vi "Basic Example.vi"   [LabVIEW 2013, in "Progress Bar.lvlib"]
uses:
  Progress Bar.lvlib
  Controls/Update Bar Actions.ctl
types:
  T1 = typedef "Progress Bar.lvlib/Update Bar Actions.ctl" = enum16{"Add To Existing", "Set to Value"}
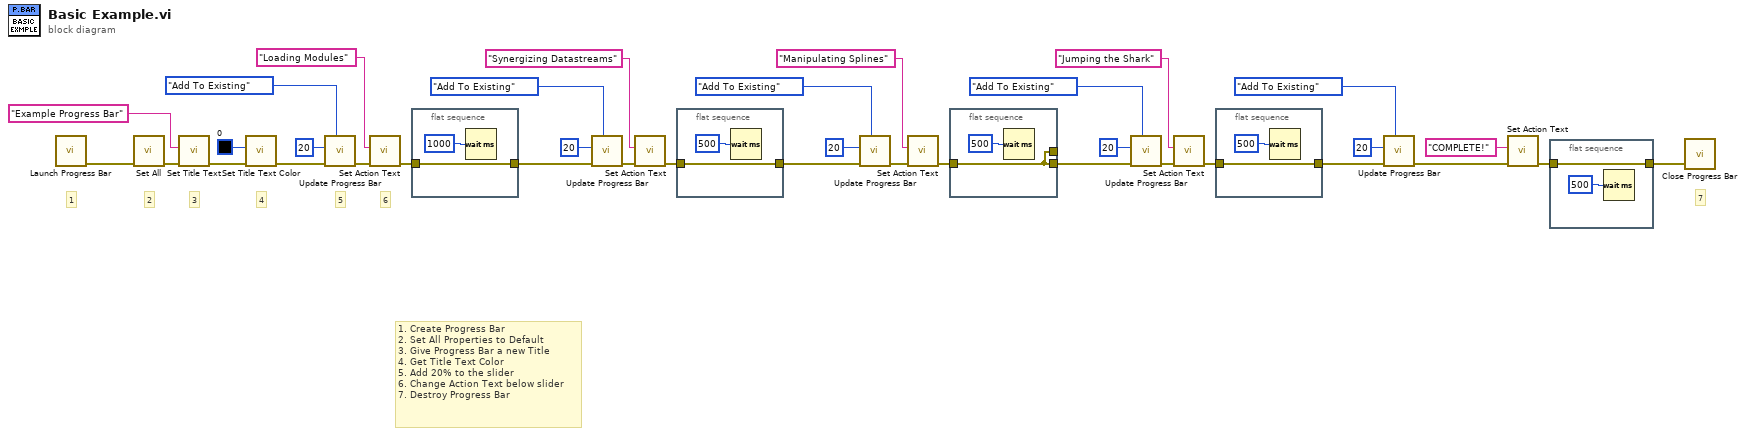
[diagram p0: block diagram]
diagram:
  # "7"
  # "6"
  # "5"
  # "4"
  # "3"
  # "2"
  # "1"
  # "1. Create Progress Bar\n2. Set All Properties to Default\n3. Give Progress Bar a new Title\n4. Get Title Text Color\n5. Add 20% to the slider\n6. Change Action Text below slider\n7. Destroy Progress Bar"
  n1 = call "Launch Progress Bar.vi"() -> ("error out"=w1:errorcluster)  [unwired: 11 in]
  n2 = call "Set All.vi"("error in (no error)"=w1) -> ("error out"=w31:errorcluster)  [unwired: 10 in]
  n3 = call "Set Title Text.vi"("error in (no error)"=w31, "Installer Title"="Example Progress Bar") -> ("error out"=w35:errorcluster)  [unwired: 9 in]
  n4 = call "Set Title Text Color.vi"("error in (no error)"=w35, "Color Box"=u32 0) -> ("error out"=w30:errorcluster)  [unwired: 9 in]
  n5 = call "Update Progress Bar.vi"("Action"=Update_Bar_Actions."Add To Existing", "error in (no error)"=w30, "Value"=u8 20) -> ("error out"=w29:errorcluster)  [unwired: 8 in]
  n6 = call "Set Action Text.vi"("error in (no error)"=w29, "Action Text"="Loading Modules") -> ("error out"=w28:errorcluster)  [unwired: 9 in]
  n7 = flat-sequence {
    tunnel: w28 -> [w37]
    tunnel: [w37] -> w12
    frame #0 {
      n8 = Wait (ms)(milliseconds to wait=u32 1000) -> ()  [unwired: 1 out]
    }
  }
  n9 = call "Update Progress Bar.vi"("Action"=Update_Bar_Actions."Add To Existing", "error in (no error)"=w12, "Value"=u8 20) -> ("error out"=w25:errorcluster)  [unwired: 8 in]
  n10 = call "Set Action Text.vi"("error in (no error)"=w25, "Action Text"="Synergizing Datastreams") -> ("error out"=w24:errorcluster)  [unwired: 9 in]
  n11 = flat-sequence {
    tunnel: w24 -> [w39]
    tunnel: [w39] -> w11
    frame #0 {
      n12 = Wait (ms)(milliseconds to wait=u32 500) -> ()  [unwired: 1 out]
    }
  }
  n13 = call "Update Progress Bar.vi"("Action"=Update_Bar_Actions."Add To Existing", "error in (no error)"=w11, "Value"=u8 20) -> ("error out"=w20:errorcluster)  [unwired: 8 in]
  n14 = call "Set Action Text.vi"("error in (no error)"=w20, "Action Text"="Manipulating Splines") -> ("error out"=w19:errorcluster)  [unwired: 9 in]
  n15 = flat-sequence {
    tunnel: w19 -> [w41]
    tunnel: [w41] -> _
    tunnel: [w41] -> w10
    frame #0 {
      n16 = Wait (ms)(milliseconds to wait=u32 500) -> ()  [unwired: 1 out]
    }
  }
  n17 = call "Update Progress Bar.vi"("Action"=Update_Bar_Actions."Add To Existing", "error in (no error)"=w10, "Value"=u8 20) -> ("error out"=w16:errorcluster)  [unwired: 8 in]
  n18 = call "Set Action Text.vi"("error in (no error)"=w16, "Action Text"="Jumping the Shark") -> ("error out"=w15:errorcluster)  [unwired: 9 in]
  n19 = flat-sequence {
    tunnel: w15 -> [w43]
    tunnel: [w43] -> w3
    frame #0 {
      n20 = Wait (ms)(milliseconds to wait=u32 500) -> ()  [unwired: 1 out]
    }
  }
  n21 = call "Update Progress Bar.vi"("Action"=Update_Bar_Actions."Add To Existing", "error in (no error)"=w3, "Value"=u8 20) -> ("error out"=w7:errorcluster)  [unwired: 8 in]
  n22 = call "Set Action Text.vi"("error in (no error)"=w7, "Action Text"="COMPLETE!") -> ("error out"=w6:errorcluster)  [unwired: 9 in]
  n23 = flat-sequence {
    tunnel: w6 -> [w45]
    tunnel: [w45] -> w2
    frame #0 {
      n24 = Wait (ms)(milliseconds to wait=u32 500) -> ()  [unwired: 1 out]
    }
  }
  n25 = call "Close Progress Bar.vi"("error in (no error)"=w2) -> ()  [unwired: 10 in, 1 out]
